vi "fpga CHOPPER TEST.vi"() -> ()   [LabVIEW 2009]
uses:
  <vilib>/eio/EIONode/EIONode.xnode
  <vilib>/rvi/eio/nirviEIOImplementation/nirviEIOImplementation.xnode
  <vilib>/rvi/eio/common/nirviEmuTemplateMethod_noerrors.vi
  <vilib>/rvi/eio/common/nirviEmuClasses.ctl
panel:
  in  "Mod7/DIO0 2":bool
  out "Mod7/DIO0":bool
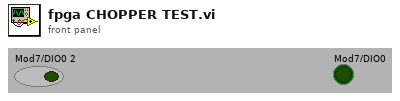
[diagram p1: front panel]
types:
  T1 = typedef "nirviEmuClasses.ctl" = enum16{"IO Read", "IO Write", "Method", "Property Read", "Property Write"}
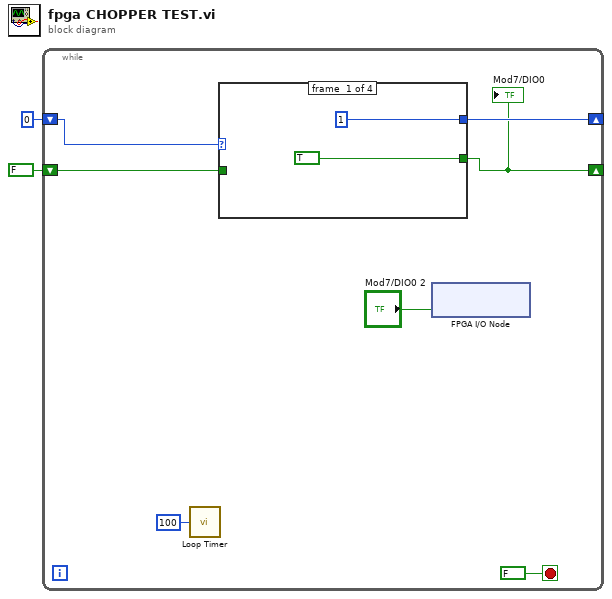
[diagram p0: block diagram]
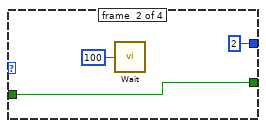
[diagram p2: hidden frame]
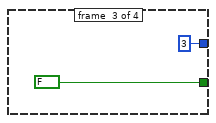
[diagram p3: hidden frame]
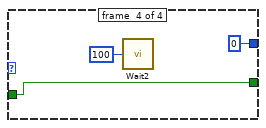
[diagram p4: hidden frame]
diagram:
  n1 = while {
    shift-right: [w8] -> _
    shift-left: i16 0 -> [w7]
    shift-right: [w4] -> _
    shift-left: FALSE ("Mod7/DIO0") -> [w6]
    stop <- FALSE stop-if-true
    n2 = call "Loop Timer"("Count(Ticks)"=u32 100) -> ()  [unwired: 1 out]
    n3 = case shown="3" w7 {
      tunnel: [TRUE ("Mod7/DIO0") w24 FALSE ("Mod7/DIO0") w29] -> w4
      tunnel: [i16 1 i16 2 i16 3 i16 0] -> w8
      tunnel: w6 -> [_ w24 _ w29]
      frame #0 {
      }
      frame #1 {
        n4 = call "Wait"("Count(mSec)"=u32 100) -> ()  [unwired: 1 out]
      }
      frame #2 {
      }
      frame #3 {
        n5 = call "Wait2"("Count(mSec)"=u32 100) -> ()  [unwired: 1 out]
      }
    }
    "Mod7/DIO0" <- w4
    n6 = xnode "FPGA I/O Node"("Mod7/DIO0"="Mod7/DIO0 2") -> ()  [unwired: 1 in, 1 out]
  }
